vi "DSF.Engine.Transfer Group.Set Timing.vi"(10 "Timing":refnum<class "Engine Timing.lvclass">, 11 "Transfer Group in":refnum<class "DSF.Engine.Transfer Group.lvclass">) -> (3 "Transfer Group out":refnum<class "DSF.Engine.Transfer Group.lvclass">)   [LabVIEW 2017, in "Data Sharing Framework Engine.lvlib" / "DSF.Engine.Transfer Group.lvclass"]
uses:
  DSF.Engine.Transfer Group.lvclass
  Source/Data Sharing Framework Core/Engine/Timing/Engine Timing.lvclass
  DSF.Engine.Transfer Group.lvclass/DSF.Engine.Transfer Group.ctl
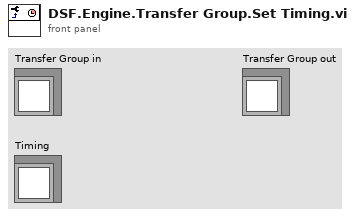
[diagram p1: front panel]
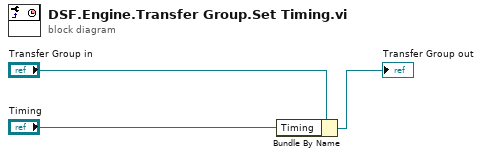
[diagram p0: block diagram]
diagram:
  n1 = Bundle By Name(cluster="Transfer Group in", "Timing"="Timing") -> (→"Transfer Group out":refnum<class "DSF.Engine.Transfer Group.lvclass">)
